vi "Pointer.Write (SGL).vi"(8 "error in (no error)":errorcluster, 10 "value":sgl, 11 "pointer in":u64) -> (0 "error out":errorcluster, 2 "value out":sgl, 3 "pointer out":u64)   [LabVIEW 2016, in "VeriStand Data.lvlib"]
doc: "Writes the contents of the provided <B>value</B> to the memory location specified by <B>pointer</B>."
uses:
  VeriStand Data.lvlib
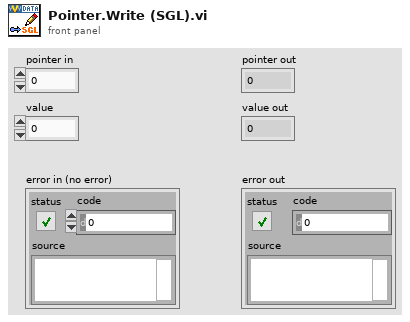
[diagram p1: front panel]
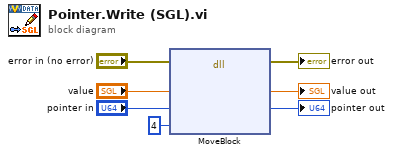
[diagram p0: block diagram]
diagram:
  n1 = dll-call lib="LabVIEW" fn="MoveBlock"(error in="error in (no error)", "ps"="value", "pd"="pointer in", "size"=4) -> (error out=→"error out":errorcluster, "ps"=→"value out":sgl, "pd"=→"pointer out":u64)  [unwired: 4 in, 1 out]
